vi "AsyncBluetoothHandler.vi"(11 "Queue":refnum<queue>) -> ()   [LabVIEW 2013, in "main.lvlib"]
uses:
  main.lvlib
  Controls/Enum Save Action Events.ctl
  C:/Users/Simon/SkyDrive/LabView/2013/DM2020/bin/medimatic_bt_receiver.dll
  bin/medimatic_bt_receiver.dll
panel:
  out "Present (s)":dbl
  out "Elapsed Time (s)":dbl
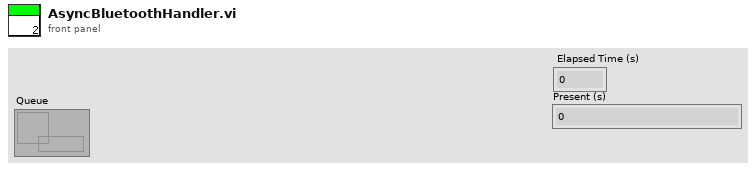
[diagram p1: front panel]
types:
  T1 = typedef "main.lvlib/Enum Save Action Events.ctl" = enum16{"LoadReportPath", "SaveReportPath", "Load Graph Path", "Save Graph Path", "LoadDataPath", "SaveDataPath", "Load Template Path", "Save Template Path", "Load PressureFactor", "Save PressureFactor", "Init", "Load Listbox", "Save Listbox", "LoadHospInfo", "SaveHospInfo", "Load DICOM Activation", "Save DICOM Activation", "LoadDICOMInfoWL", "SaveDICOMInfoWL", "LoadDICOMInfoPACS", "SaveDICOMInfoPACS", "Load ArmCalcMethod", "Save ArmCalcMethod", "LoadItemTags", "SaveItemTags", "LoadDICOMEncoding", "SaveDICOMEncoding", "LoadJournalType", "SaveJournalType", "LoadAcqFilterType", "SaveAcqFilterType", "Load Sequence", "Save Sequence", "Load Acquisition Mode", "Save Acquisition Mode", "Load General Settings", "Save General Settings", "Load Language", "Save Language", "Load Dicom Tags", "Save Dicom Tags", "Load BT Serial", "Save BT Serial", "Load BT License", "Save BT License"}
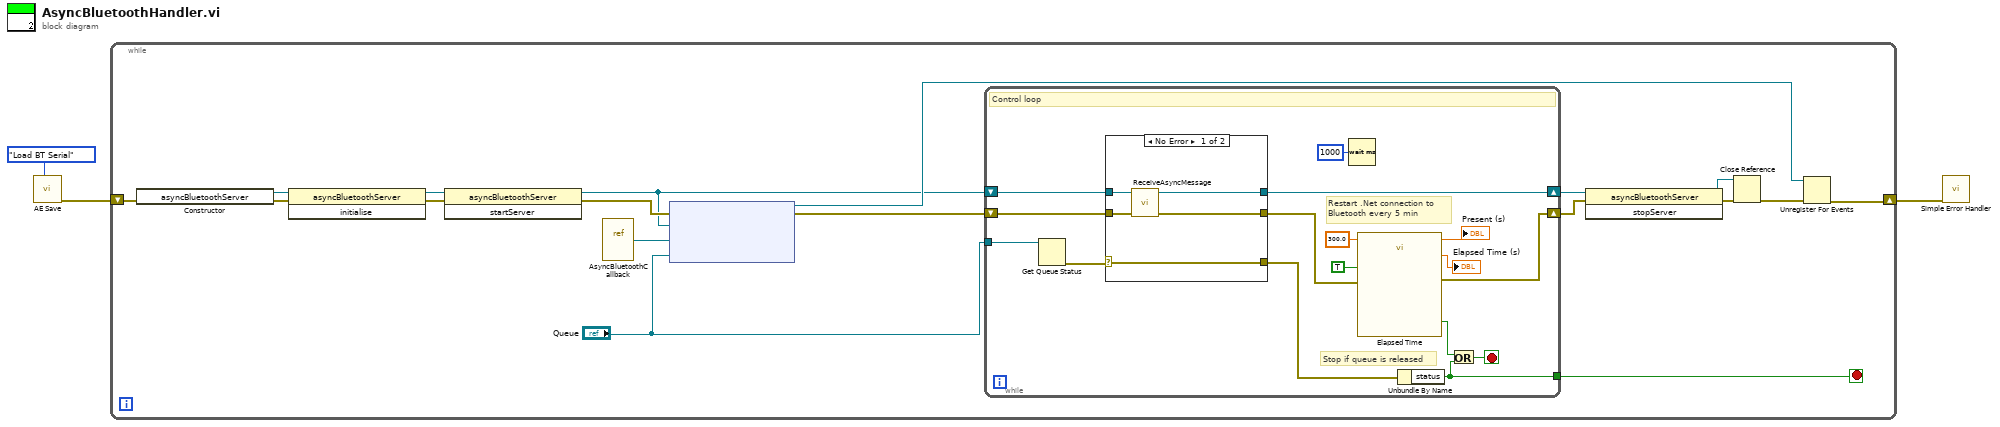
[diagram p0: block diagram]
diagram:
  n1 = call "AE Save.vi"("Action"=Enum_Save_Action_Events."Load BT Serial") -> ("error out"=w2:errorcluster)  [unwired: 8 in, 1 out]
  n2 = while {
    shift-right: [w8] -> w1
    shift-left: w2 -> [w14]
    stop <- w13 stop-if-true
    n3 = constructor class="asyncBluetoothServer"(error in=w14) -> (reference out=w21:refnum<k24>, error out=w19:errorcluster)  [unwired: 2 in, 1 out]
    n4 = invoke class="asyncBluetoothServer" method="initialise"(reference=w21, error in=w19) -> (reference out=w20:refnum<k24>, error out=w18:errorcluster)  [unwired: 1 in, 1 out]
    n5 = invoke class="asyncBluetoothServer" method="startServer"(reference=w20, error in=w18) -> (reference out=w5:refnum<k24>, error out=w11:errorcluster)  [unwired: 1 in, 1 out]
    n6 = vi-ref "AsyncBluetoothCallback.vi"() -> ("vi reference"=w4:refnum<vi>)
    n7 = node(w11, w5, w4, "Queue") -> (w7:refnum<k27>, w10:errorcluster)  [unwired: 1 in]
    n8 = while {
      tunnel: "Queue" -> [w33]
      shift-right: [w36] -> w15
      shift-left: w5 -> [w37]
      shift-right: [w30] -> w12
      shift-left: w10 -> [w35]
      tunnel: [w24] -> w13
      stop <- w27 stop-if-true
      # "Restart .Net connection to\nBluetooth every 5 min"
      # "Stop if queue is released"
      # "Control loop"
      n9 = Get Queue Status(queue=w33) -> (error out=w32:errorcluster)  [unwired: 2 in, 7 out]
      n10 = case shown="No Error" w32 {
        selector: w32 -> [w42 w45]
        tunnel: w37 -> [w41 w44]
        tunnel: [w39 w44] -> w36
        tunnel: w35 -> [w40 w43]
        tunnel: [w38 w43] -> w31
        tunnel: [w42 w45] -> w25
        frame No Error {
          n11 = call "ReceiveAsyncMessage.vi"("error in (no error)"=w40, "reference input"=w41) -> ("error out"=w38:errorcluster, "reference output"=w39:refnum<k24>)  [unwired: 8 in]
        }
        frame Error {
        }
      }
      n12 = Wait (ms)(milliseconds to wait=1000) -> ()  [unwired: 1 out]
      n13 = call "Elapsed Time"("Time Target (s)"=300.0, "Auto Reset"=TRUE, "error in (no error)"=w31) -> ("Present (s)"=→"Present (s)":dbl, "Elapsed Time (s)"=→"Elapsed Time (s)":dbl, "Time has Elapsed"=w26:bool, "error out"=w30:errorcluster)  [unwired: 9 in, 4 out]
      n14 = Unbundle By Name(w25) -> ("status"=w24:bool)
      n15 = Or(x=w26, y=w24) -> (x .or. y?=w27:bool)
    }
    n16 = invoke class="asyncBluetoothServer" method="stopServer"(reference=w15, error in=w12) -> (reference out=w16:refnum<k24>, error out=w17:errorcluster)  [unwired: 1 in, 1 out]
    n17 = Close Reference(reference=w16, error in (no error)=w17) -> (error out=w9:errorcluster)
    n18 = Unregister For Events(event registration refnum=w7, error in=w9) -> (error out=w8:errorcluster)
  }
  n19 = call <vilib>:"Simple Error Handler.vi"("error in (no error)"=w1) -> ()  [unwired: 4 in, 5 out]
